vi "Heat2D_X Dirichlet Type.vi"(7 "Left?":bool=TRUE, 8 "step (n+1)":i32, 9 "Boundary Condition":cluster{"type":T1, "Value":dbl[][]}[](array[cluster]) {"type" items=["Dirichlet", "Neumann"]}, 10 "Coefficients":T2, 11 "BC Value":dbl[](array[numeric])) -> (3 "U":dbl[](array[numeric]))   [LabVIEW 2020, in "NI_PDE.lvlib"]
uses:
  <vilib>/gmath/NI_PDE.lvlib
  <vilib>/gmath/pde.llb/Common/PDE_BC Type.ctl
  <vilib>/Analysis/2dsp.llb/1D Convolution (DBL).vi
  <vilib>/Analysis/NI_AALPro.lvlib
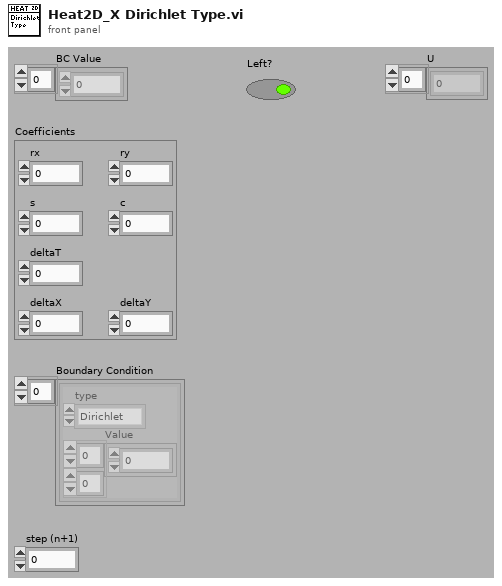
[diagram p1: front panel]
types:
  T1 = typedef "NI_PDE.lvlib/PDE_BC Type.ctl" = i32
  T2 = cluster{"rx":dbl, "ry":dbl, "s":dbl, "c":dbl, "deltaT":dbl, "deltaX":dbl, "deltaY":dbl}
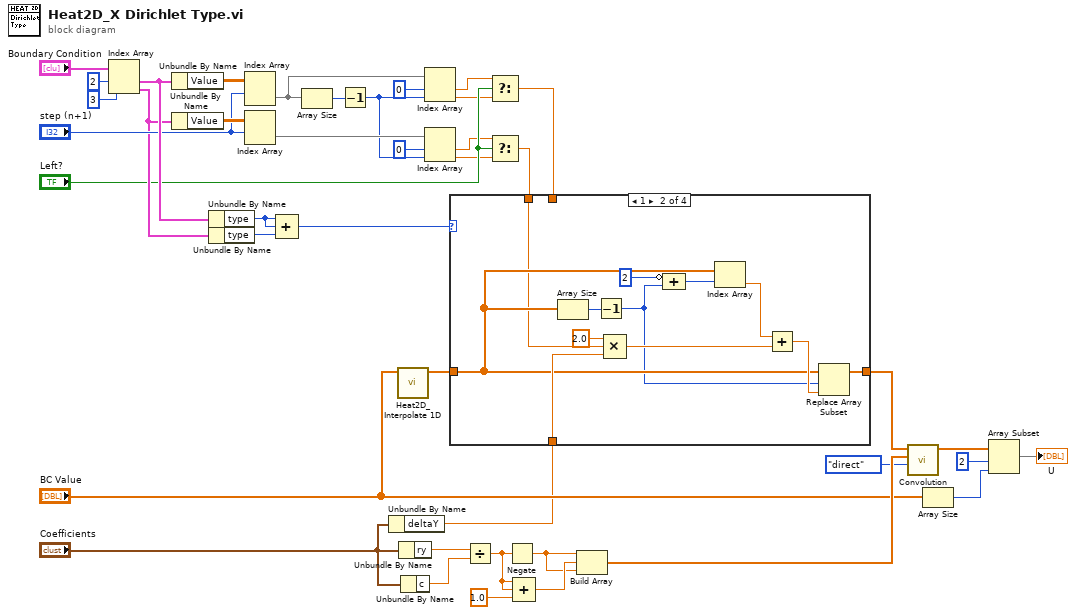
[diagram p0: block diagram]
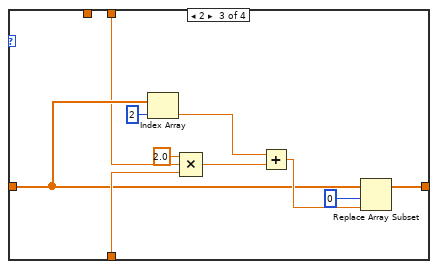
[diagram p3: hidden frame]
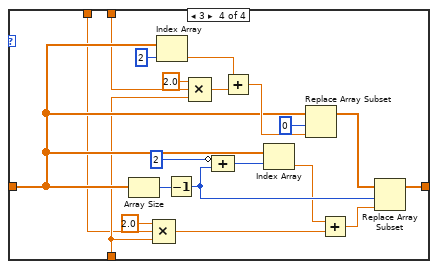
[diagram p4: hidden frame]
diagram:
  n1 = Index Array(array="Boundary Condition", index #1=2 ("index"), index #2=3 ("index")) -> (element #1=w25:cluster{"type":T1, "Value":dbl[][]}, element #2=w20:cluster{"type":T1, "Value":dbl[][]})
  n2 = Unbundle By Name(w25) -> ("Value"=w24:dbl[][])
  n3 = Unbundle By Name(w20) -> ("Value"=w23:dbl[][])
  n4 = Unbundle By Name(w25) -> ("type"=w27:T1)
  n5 = Unbundle By Name(w20) -> ("type"=w26:T1)
  n6 = Index Array(array=w24, index (row)="step (n+1)") -> (element=w14:dbl[])  [unwired: 1 in]
  n7 = Index Array(array=w23, index (row)="step (n+1)") -> (element=w16:dbl[])  [unwired: 1 in]
  n8 = Compound Arithmetic op=ADD(w27, w27, w26) -> (w17:T1)
  n9 = Array Size(array=w14) -> (size(s)=w13:i32)
  n10 = Decrement(x=w13) -> (x-1=w12:i32)
  n11 = Unbundle By Name("Coefficients") -> ("deltaY"=w3:dbl)
  n12 = call <vilib>:"Heat2D_Interpolate 1D.vi"("X"="BC Value") -> ("Interp(X)"=w4:dbl[])  [unwired: 1 in, 9 out]
  n13 = Unbundle By Name("Coefficients") -> ("ry"=w18:dbl)
  n14 = Unbundle By Name("Coefficients") -> ("c"=w36:dbl)
  n15 = Index Array(array=w14, index #1=0 ("index"), index #2=w12) -> (element #1=w9:dbl, element #2=w6:dbl)
  n16 = Index Array(array=w16, index #1=0 ("index"), index #2=w12) -> (element #1=w8:dbl, element #2=w7:dbl)
  n17 = Divide(x=w18, y=w36) -> (x/y=w40:dbl)
  n18 = Select(t=w9, s="Left?", f=w6) -> (s? t:f=w5:dbl)
  n19 = Select(t=w8, s="Left?", f=w7) -> (s? t:f=w2:dbl)
  n20 = case shown="1" w17 {
    tunnel: w4 -> [w42 w49 w56 w69]
    tunnel: [w42 w44 w62 w76] -> w1
    tunnel: w3 -> [_ w54 w64 w68]
    tunnel: w5 -> [_ _ w55 w65]
    tunnel: w2 -> [_ w43 _ w66]
    frame 0, Default {
    }
    frame 1 {
      n21 = Array Size(array=w49) -> (size(s)=w52:i32)
      n22 = Decrement(x=w52) -> (x-1=w48:i32)
      n23 = Compound Arithmetic op=MULTIPLY(2.0 ("value"), w43, w54) -> (w51:dbl)
      n24 = Compound Arithmetic op=ADD(invert 2 ("y"), w48) -> (w46:i32)
      n25 = Index Array(array=w49, index=w46) -> (element=w45:dbl)
      n26 = Add(x=w45, y=w51) -> (x+y=w50:dbl)
      n27 = Replace Array Subset(array=w49, new element=w50, index=w48) -> (w44:dbl[])
    }
    frame 2 {
      n28 = Index Array(array=w56, index=2) -> (element=w58:dbl)
      n29 = Compound Arithmetic op=MULTIPLY(2.0 ("value"), w55, w64) -> (w61:dbl)
      n30 = Add(x=w58, y=w61) -> (x+y=w60:dbl)
      n31 = Replace Array Subset(array=w56, new element=w60, index=0) -> (w62:dbl[])
    }
    frame 3 {
      n32 = Array Size(array=w69) -> (size(s)=w83:i32)
      n33 = Compound Arithmetic op=MULTIPLY(2.0 ("value"), w66, w68) -> (w82:dbl)
      n34 = Index Array(array=w69, index=2) -> (element=w71:dbl)
      n35 = Decrement(x=w83) -> (x-1=w80:i32)
      n36 = Compound Arithmetic op=MULTIPLY(2.0 ("value"), w65, w68) -> (w74:dbl)
      n37 = Compound Arithmetic op=ADD(invert 2 ("y"), w80) -> (w78:i32)
      n38 = Add(x=w71, y=w74) -> (x+y=w73:dbl)
      n39 = Index Array(array=w69, index=w78) -> (element=w77:dbl)
      n40 = Replace Array Subset(array=w69, new element=w73, index=0) -> (w67:dbl[])
      n41 = Add(x=w77, y=w82) -> (x+y=w81:dbl)
      n42 = Replace Array Subset(array=w67, new element=w81, index=w80) -> (w76:dbl[])
    }
  }
  n43 = Negate(x=w40) -> (-x=w37:dbl)
  n44 = Compound Arithmetic op=ADD(w40, w40, 1.0 ("value")) -> (w38:dbl)
  n45 = Build Array(w37, w38, w37) -> (w41:dbl[])
  n46 = call-poly <vilib>:"Convolution.vi"("algorithm"=enum32{"direct", "frequency domain"}."direct", "Y"=w41, "X"=w1) -> ("X * Y"=w34:dbl[])  [unwired: 8 out]
  n47 = Array Size(array="BC Value") -> (size(s)=w33:i32)
  n48 = Array Subset(array=w34, index=2, length=w33) -> (→"U":dbl[])
